vi "DB测试.vi"() -> ()   [LabVIEW 2017]
panel:
  in  "value":u16
  out "Content":u16
  in  "DB5000.W":string[](array[string])=["DB5000.228"]
  out "添加的数组":sgl[](array[numeric])=[0.030381944, 0.03436053, 0.033275463, 0.05389178, 0.033998843, 0.03436053, 0.03725405, 3.0110676, 0.036892362, 0.041232638, 0.96571183]
  in  "DB5000.R":string[](array[string])=["DB5000.136", "DB5000.140", "DB5000.144", "DB5000.148", "DB5000.152", "DB5000.156", "DB5000.160", "DB5000.164", "DB5000.168", "DB5000.172", "DB5000.176"]
  out "IO":T1={"字符识别启动信号-读"=FALSE, "电脑1扫码枪\n触发-读"=FALSE, "电脑1CCD读取\n字符触发-读"=FALSE, "电脑1表面检测\n触发-读"=FALSE, "电脑1穿管检测\n触发-读"=TRUE, "区间位置1-读"=FALSE, "区间位置2-读"=FALSE, "区间位置3-读"=FALSE, "区间位置4-读"=FALSE, "区间位置5-读"=FALSE, "区间位置6-读"=FALSE, "区间位置7-读"=FALSE, "区间位置8-读"=FALSE, "区间位置9-读"=FALSE, "区间位置10-读"=FALSE, "区间位置11-读"=FALSE, "区间位置12-读"=FALSE, "区间位置13-读"=FALSE, "区间位置14-读"=FALSE, "区间位置15-读"=FALSE, "区间位置16-读"=FALSE, "区间位置17-读"=FALSE, "区间位置18-读"=FALSE, "区间位置19-读"=FALSE, "夹爪1状态-读"=FALSE, "夹爪2状态-读"=FALSE, "夹爪3状态-读"=FALSE, "夹爪4状态-读"=FALSE, "夹爪5状态-读"=FALSE, "夹爪6状态-读"=FALSE, "电脑1压力获取\n触发-读"=TRUE, "电脑1产品前后位置\n切换触发-读"=FALSE, "夹爪10状态-读"=FALSE, "夹爪9状态-读"=FALSE, "夹爪8状态-读"=FALSE, "夹爪7状态-读"=FALSE, "PC1 ready-写 "=TRUE, "混料-写"=TRUE, "字符1检测pass-写"=TRUE, "字符1检测fail-写"=TRUE, "表面检测pass-写"=TRUE, "表面检测fail-写"=TRUE, "穿管检测pass-写"=TRUE, "穿管检测fail-写"=TRUE, "扫码枪pass-写"=TRUE, "扫码枪fail-写"=TRUE, "产品尺寸A-写"=TRUE, "产品尺寸B-写"=TRUE, "数据传递信号-读"=TRUE, "表面检测完成信号-读"=TRUE, "穿管NG停止信号-写"=TRUE, "电脑1返工信号-写"=TRUE, "PLC初始化信号-读"=TRUE, "产品尺寸C-写"=TRUE, "表面检测错位气缸-读"=TRUE, "电脑1衬丝检测触发-读"=TRUE, "衬丝能检测pass-写"=TRUE, "衬丝能检测fail-写"=TRUE, "长衬丝-写"=TRUE, "短衬丝-写"=TRUE, "细料-写"=TRUE, "粗料-写"=TRUE, "一致性检测触发-读"=TRUE}
  out "数值":i32=288
  out "IsSuccess 3":bool
  out "组合框":string(combo)="DB5000.01"
  in  "信号":bool
  out "IsSuccess 2":bool=TRUE
  in  "BD5000.X":string[](array[string])=["DB5000.00", "DB5000.100", "DB5000.101", "DB5000.102", "DB5000.103", "DB5000.104", "DB5000.105", "DB5000.106", "DB5000.107", "DB5000.108", "DB5000.109", "DB5000.110", "DB5000.111", "DB5000.112", "DB5000.113", "DB5000.114", "DB5000.115", "DB5000.116", "DB5000.117", "DB5000.118", "DB5000.119", "DB5000.120", "DB5000.121", "DB5000.122", "DB5000.123", "DB5000.124", "DB5000.125", "DB5000.126", "DB5000.127", "DB5000.128", "DB5000.129", "DB5000.130", "DB5000.131", "DB5000.132", "DB5000.133", "DB5000.134", "DB5000.200", "DB5000.201", "DB5000.202", "DB5000.203", "DB5000.204", "DB5000.205", "DB5000.206", "DB5000.207", "DB5000.208", "DB5000.209", "DB5000.210", "DB5000.211", "DB5000.212", "DB5000.213", "DB5000.214", "DB5000.215", "DB5000.216", "DB5000.217", "DB5000.218", "DB5000.219", "DB5000.220", "DB5000.221", "DB5000.222", "DB5000.223", "DB5000.225", "DB5000.226", "DB5000.227"]
  in  "停止":bool
  out "error out":errorcluster caption="错误输出"
  out "结果数组":bool[](array[boolean])=[FALSE, FALSE, FALSE, FALSE, TRUE, FALSE, FALSE, FALSE, FALSE, FALSE, FALSE, FALSE, FALSE, FALSE, FALSE, FALSE, FALSE, FALSE, FALSE, FALSE, FALSE, FALSE, FALSE, FALSE, FALSE, FALSE, FALSE, FALSE, FALSE, FALSE, FALSE, FALSE, FALSE, FALSE, TRUE, FALSE, TRUE, TRUE, TRUE, TRUE, TRUE, TRUE, TRUE, TRUE, TRUE, TRUE, TRUE, TRUE, TRUE, TRUE, TRUE, TRUE, TRUE, TRUE, TRUE, TRUE, TRUE, TRUE, TRUE, TRUE, TRUE, TRUE, TRUE]
  out "IsSuccess":bool=TRUE
  out "通讯状态":bool=TRUE
  in  "错误输入（无错误）":errorcluster
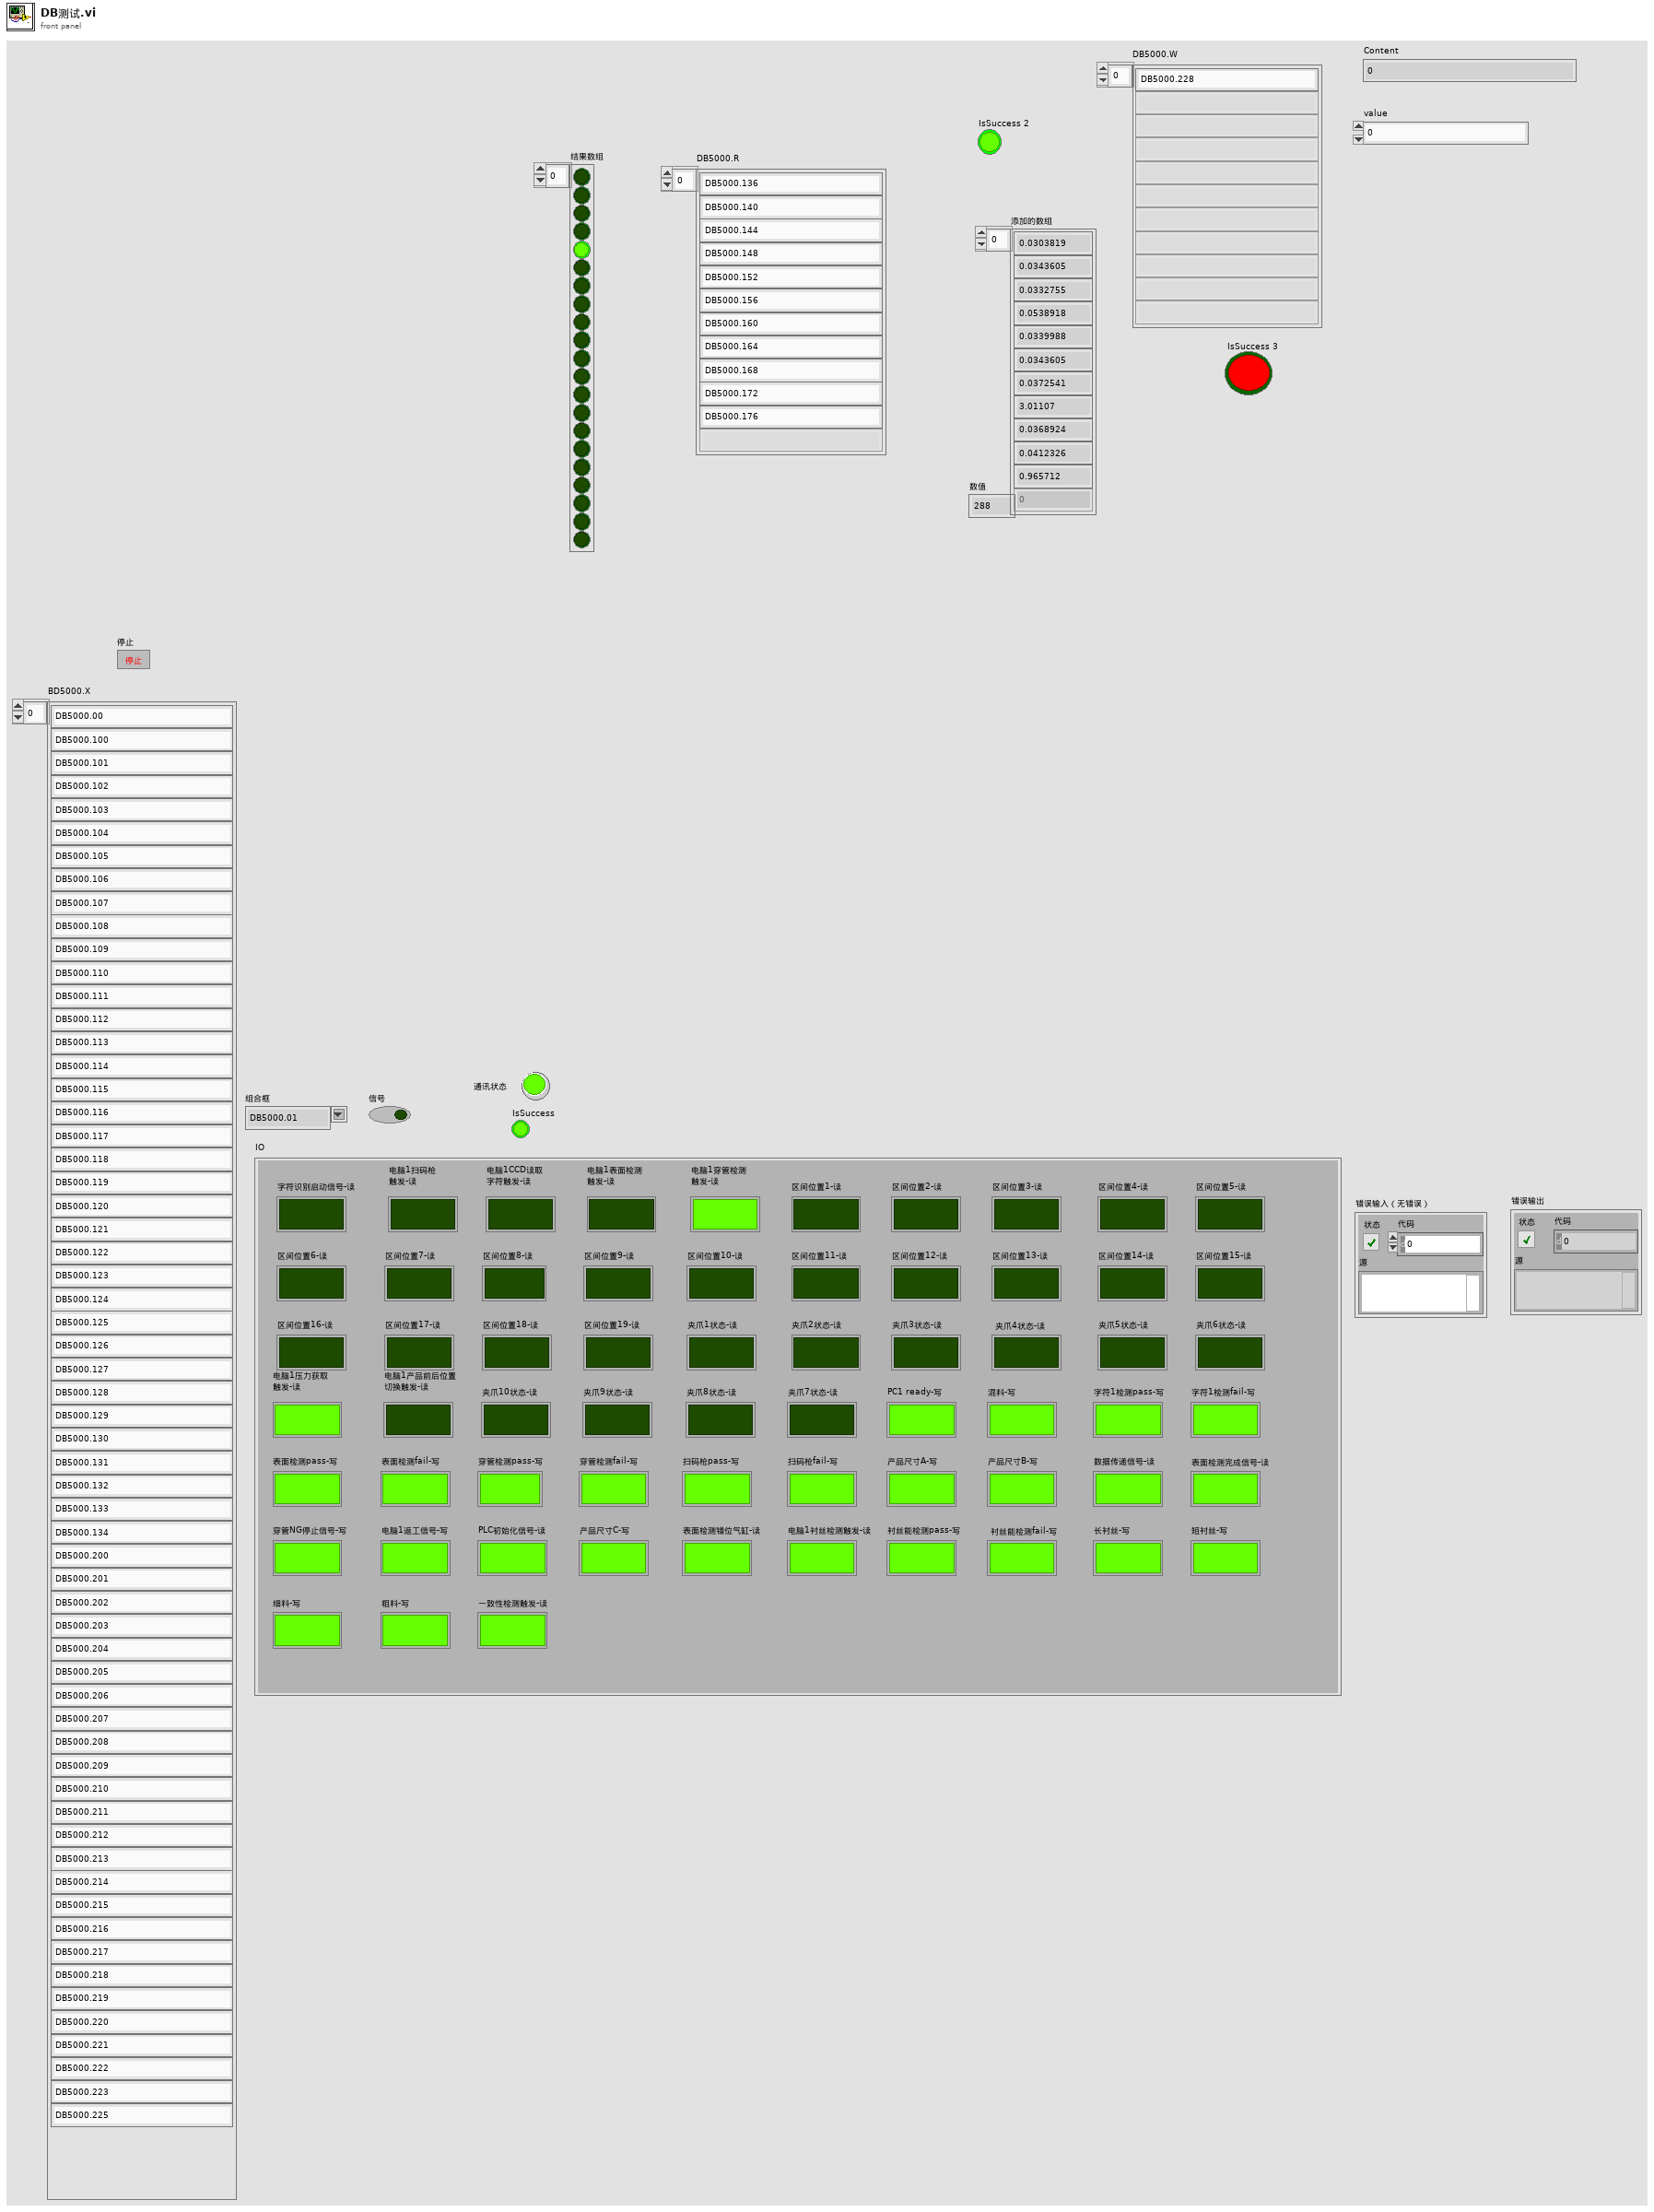
[diagram p1: front panel]
types:
  T1 = cluster{"字符识别启动信号-读":bool, "电脑1扫码枪\n触发-读":bool, "电脑1CCD读取\n字符触发-读":bool, "电脑1表面检测\n触发-读":bool, "电脑1穿管检测\n触发-读":bool, "区间位置1-读":bool, "区间位置2-读":bool, "区间位置3-读":bool, "区间位置4-读":bool, "区间位置5-读":bool, "区间位置6-读":bool, "区间位置7-读":bool, "区间位置8-读":bool, "区间位置9-读":bool, "区间位置10-读":bool, "区间位置11-读":bool, "区间位置12-读":bool, "区间位置13-读":bool, "区间位置14-读":bool, "区间位置15-读":bool, "区间位置16-读":bool, "区间位置17-读":bool, "区间位置18-读":bool, "区间位置19-读":bool, "夹爪1状态-读":bool, "夹爪2状态-读":bool, "夹爪3状态-读":bool, "夹爪4状态-读":bool, "夹爪5状态-读":bool, "夹爪6状态-读":bool, "电脑1压力获取\n触发-读":bool, "电脑1产品前后位置\n切换触发-读":bool, "夹爪10状态-读":bool, "夹爪9状态-读":bool, "夹爪8状态-读":bool, "夹爪7状态-读":bool, "PC1 ready-写 ":bool, "混料-写":bool, "字符1检测pass-写":bool, "字符1检测fail-写":bool, "表面检测pass-写":bool, "表面检测fail-写":bool, "穿管检测pass-写":bool, "穿管检测fail-写":bool, "扫码枪pass-写":bool, "扫码枪fail-写":bool, "产品尺寸A-写":bool, "产品尺寸B-写":bool, "数据传递信号-读":bool, "表面检测完成信号-读":bool, "穿管NG停止信号-写":bool, "电脑1返工信号-写":bool, "PLC初始化信号-读":bool, "产品尺寸C-写":bool, "表面检测错位气缸-读":bool, "电脑1衬丝检测触发-读":bool, "衬丝能检测pass-写":bool, "衬丝能检测fail-写":bool, "长衬丝-写":bool, "短衬丝-写":bool, "细料-写":bool, "粗料-写":bool, "一致性检测触发-读":bool}
  T2 = cluster{"字符识别启动信号-读":bool, "电脑1扫码枪\n触发-读":bool, "电脑1CCD读取\n字符触发-读":bool, "电脑1表面检测\n触发-读":bool, "电脑1穿管检测\n触发-读":bool, "区间位置1-读":bool, "区间位置2-读":bool, "区间位置3-读":bool, "区间位置4-读":bool, "区间位置5-读":bool, "区间位置6-读":bool, "区间位置7-读":bool, "区间位置8-读":bool, "区间位置9-读":bool, "区间位置10-读":bool, "区间位置11-读":bool, "区间位置12-读":bool, "区间位置13-读":bool, "区间位置14-读":bool, "区间位置15-读":bool, "区间位置16-读":bool, "区间位置17-读":bool, "区间位置18-读":bool, "区间位置19-读":bool, "夹爪1状态-读":bool, "夹爪2状态-读":bool, "夹爪3状态-读":bool, "夹爪4状态-读":bool, "夹爪5状态-读":bool, "夹爪6状态-读":bool, "夹爪7状态-读":bool, "夹爪8状态-读":bool, "夹爪9状态-读":bool, "夹爪10状态-读":bool, "电脑1产品前后位置\n切换触发-读":bool, "电脑1压力获取\n触发-读":bool, "PC1 ready-写 ":bool, "混料-写":bool, "字符1检测pass-写":bool, "字符1检测fail-写":bool, "表面检测pass-写":bool, "表面检测fail-写":bool, "穿管检测pass-写":bool, "穿管检测fail-写":bool, "扫码枪pass-写":bool, "扫码枪fail-写":bool, "产品尺寸A-写":bool, "产品尺寸B-写":bool, "数据传递信号-读":bool, "表面检测完成信号-读":bool, "穿管NG停止信号-写":bool, "电脑1返工信号-写":bool, "PLC初始化信号-读":bool, "产品尺寸C-写":bool, "表面检测错位气缸-读":bool, "电脑1衬丝检测触发-读":bool, "衬丝能检测pass-写":bool, "衬丝能检测fail-写":bool, "长衬丝-写":bool, "短衬丝-写":bool, "细料-写":bool, "粗料-写":bool, "一致性检测触发-读":bool}
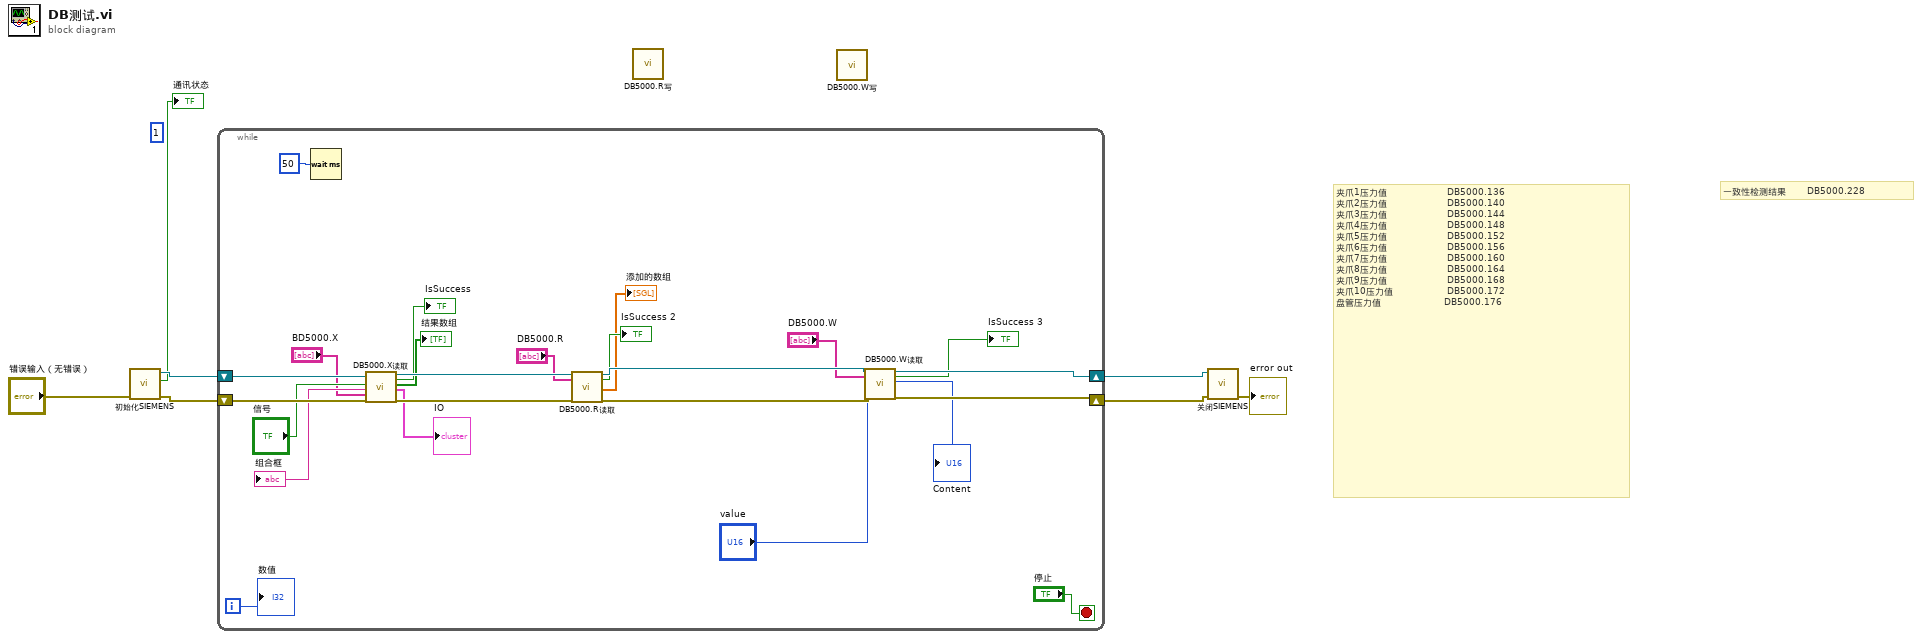
[diagram p0: block diagram]
diagram:
  (unwired) 1
  # "一致性检测结果       DB5000.228"
  # "夹爪1压力值                    DB5000.136\n夹爪2压力值                    DB5000.140\n夹爪3压力值                    DB5000.144\n夹爪4压力值                    DB5000.148\n夹爪5压力值                    DB5000.152\n夹爪6压力值                    DB5000.156\n夹爪7压力值                    DB5000.160\n夹爪8压力值                    DB5000.164\n夹爪9压力值                    DB5000.168\n夹爪10压力值                  DB5000.172\n盘管压力值                     DB5000.176"
  n1 = call "初始化SIEMENS.vi"("错误输入（无错误）"="错误输入（无错误）") -> ("错误输出"=w4:errorcluster, "通讯状态"=→"通讯状态":bool, "gInitialSIEMENSS7"=w6:refnum<k24>)  [unwired: 8 in]
  n2 = while {
    shift-right: [w28] -> w3
    shift-left: w6 -> [w25]
    shift-right: [w29] -> w2
    shift-left: w4 -> [w30]
    i -> [w27]
    stop <- "停止" stop-if-true
    n3 = Wait (ms)(milliseconds to wait=u32 50 ("等待时间（毫秒）")) -> ()  [unwired: 1 out]
    n4 = call "DB5000.X读取.vi"("gInitialSIEMENSS7 In"=w25, "字符识别NG信号"="信号", "地址数组 2"="BD5000.X", "error in (no error)"=w30) -> ("组合框"=→"组合框":string, "gInitialSIEMENSS7 Out"=w19:refnum<k24>, "IsSuccess"=→"IsSuccess":bool, "结果数组"=→"结果数组":bool[], "IO"=→"IO":T2, "error out"=w18:errorcluster)  [unwired: 10 in]
    n5 = call "DB5000.R读取.vi"("gInitialSIEMENSS7 In"=w19, "地址数组"="DB5000.R", "error in (no error)"=w18) -> ("gInitialSIEMENSS7 Out"=w24:refnum<k24>, "IsSuccess"=→"IsSuccess 2":bool, "添加的数组"=→"添加的数组":sgl[], "error out"=w23:errorcluster)  [unwired: 13 in]
    n6 = call "DB5000.W读取.vi"("gInitialSIEMENSS7 In"=w24, "地址数组"="DB5000.W", "value"="value", "error in (no error)"=w23) -> ("gInitialSIEMENSS7 Out"=w28:refnum<k24>, "IsSuccess"=→"IsSuccess 3":bool, "Content"=→"Content":u16, "error out"=w29:errorcluster)  [unwired: 12 in]
    "数值" <- w27
  }
  n7 = call "DB5000.R写.vi"() -> ()  [unwired: 16 in, 4 out]
  n8 = call "DB5000.W写.vi"() -> ()  [unwired: 16 in, 4 out]
  n9 = call "关闭SIEMENS.vi"("error in (no error)"=w2, "gInitialSIEMENSS7 In"=w3) -> ("error out"=→"error out":errorcluster)  [unwired: 9 in]
